vi "Subpanel - Latch Test.vi"(0 "VI Reference In":refnum<vi>, 5 "Subpanel Details":string, 11 "error in (no error)":errorcluster) -> (4 "VI Reference Out":refnum<vi>, 15 "error out":errorcluster)   [LabVIEW 2016]
uses:
  main/apis/Stimulus/KeyBoardSimulation/ValueSignalLatchBooleanString.vi
  main/apis/Assert/AssertControlValue/Equal.vi
  <vilib>/addons/_JKI Toolkits/Caraya/classes/Test/Test.lvclass
  main/Drona.lvlib
  main/apis/Assert/AssertControlValue/AssertControlValue.lvlib
  main/apis/Stimulus/KeyBoardSimulation/KeyboardSimulation.lvlib
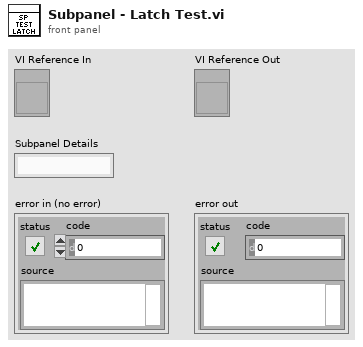
[diagram p1: front panel]
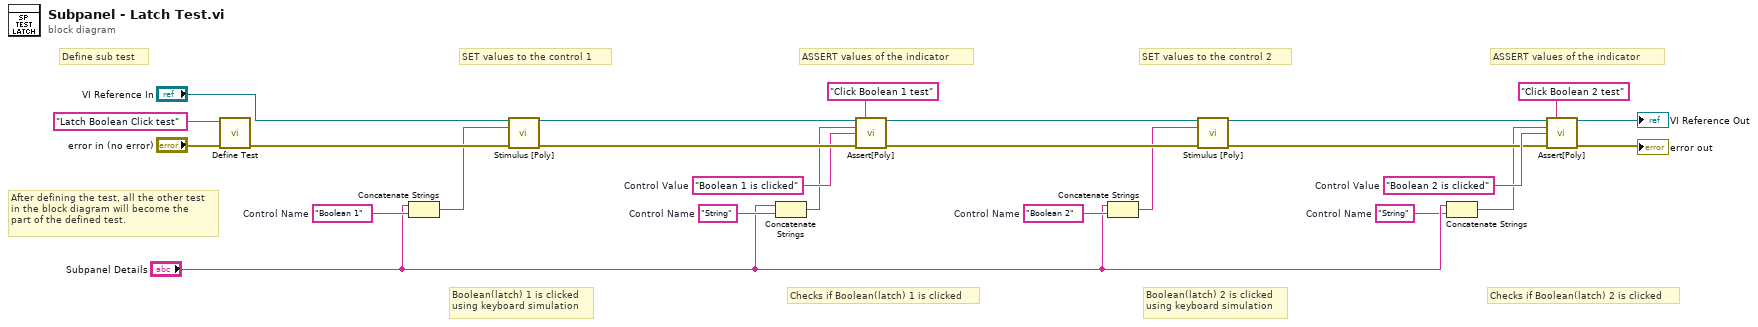
[diagram p0: block diagram]
diagram:
  w2 = "String"  # Control Name
  w19 = "Boolean 2 is clicked"  # Control Value
  w5 = "Boolean 2"  # Control Name
  w7 = "String"  # Control Name
  w22 = "Boolean 1 is clicked"  # Control Value
  w9 = "Boolean 1"  # Control Name
  # "Checks if Boolean(latch) 2 is clicked"
  # "ASSERT values of the indicator"
  # "Boolean(latch) 2 is clicked\nusing keyboard simulation"
  # "SET values to the control 2"
  # "Checks if Boolean(latch) 1 is clicked"
  # "ASSERT values of the indicator"
  # "Boolean(latch) 1 is clicked\nusing keyboard simulation"
  # "SET values to the control 1"
  # "After defining the test, all the other test\nin the block diagram will become the \npart of the defined test."
  # "Define sub test"
  n1 = call <vilib>:"Define Test.vi"("error in (no error)"="error in (no error)", "Label (VI Title)"="Latch Boolean Click test") -> ("error out"=w13:errorcluster)  [unwired: 9 in]
  n2 = Concatenate Strings("Subpanel Details", w9) -> (w8:string)
  n3 = call-poly "Stimulus [Poly].vi"("VI Reference In"="VI Reference In", "Control Path"=w8, "error in"=w13) -> ("VI Reference Out"=w23:refnum<vi>, "error out"=w24:errorcluster)  [unwired: 11 in]
  n4 = Concatenate Strings("Subpanel Details", w7) -> (w6:string)
  n5 = call-poly "Assert[Poly].vi"("VI Reference In"=w23, "Label"="Click Boolean 1 test" ("Label (VI Title)"), "Control Path"=w6, "Control Value"=w22, "Error In"=w24) -> ("VI Reference Out"=w16:refnum<vi>, "Error Out"=w17:errorcluster)  [unwired: 9 in]
  n6 = Concatenate Strings("Subpanel Details", w5) -> (w4:string)
  n7 = call-poly "Stimulus [Poly].vi"("VI Reference In"=w16, "Control Path"=w4, "error in"=w17) -> ("VI Reference Out"=w14:refnum<vi>, "error out"=w15:errorcluster)  [unwired: 11 in]
  n8 = Concatenate Strings("Subpanel Details", w2) -> (w1:string)
  n9 = call-poly "Assert[Poly].vi"("VI Reference In"=w14, "Label"="Click Boolean 2 test" ("Label (VI Title)"), "Control Path"=w1, "Control Value"=w19, "Error In"=w15) -> ("VI Reference Out"=→"VI Reference Out":refnum<vi>, "Error Out"=→"error out":errorcluster)  [unwired: 9 in]
